vi "SLMControl.vi"(8 "error in":errorcluster, 9 "Com-in":refnum<queue>, 10 "Com-out":refnum<queue>) -> (0 "error out":errorcluster)   [LabVIEW 2013, in "SLMControl.lvlib"]
uses:
  SLMControl.lvlib
  SA-SLMAPI/Sources/Message.lvclass
  Sources/Main/Status-LEDs.ctl
  Sources/Main/Options.ctl
  Sources/Main/Main-actions.ctl
  Sources/Main/Enqueue-modes.ctl
  Sources/Main/Deposition-actions.ctl
  Sources/Main/Lasing-actions.ctl
  Sources/Main/SC-Main.lvclass
  Sources/UI/SC-UI.lvclass
panel:
  in  "Clear":bool
  in  "Load configuration":bool
  in  "Abort":bool
  in  "Save configuration":bool
  in  "Activate":bool
  in  "Load deposition files":bool
  in  "Load lasing files":bool
  in  "Execute":bool
  in  "Help":bool
  in  "Options":T1
  out "Last elapsed time":dbl caption="Time [s]" format="%.2f"
  out "Current iteration":i32
  out "Current layer":i32
  out "Lasing job":string
  out "Deposition status":string
  out "Status LEDs":T2 caption="Status"
  in  "Files":i32(listbox)
  out "Status":string caption="Status:"
  out "Action":string caption="Action:"
  # "Config"
  # "Exec"
  # "Files"
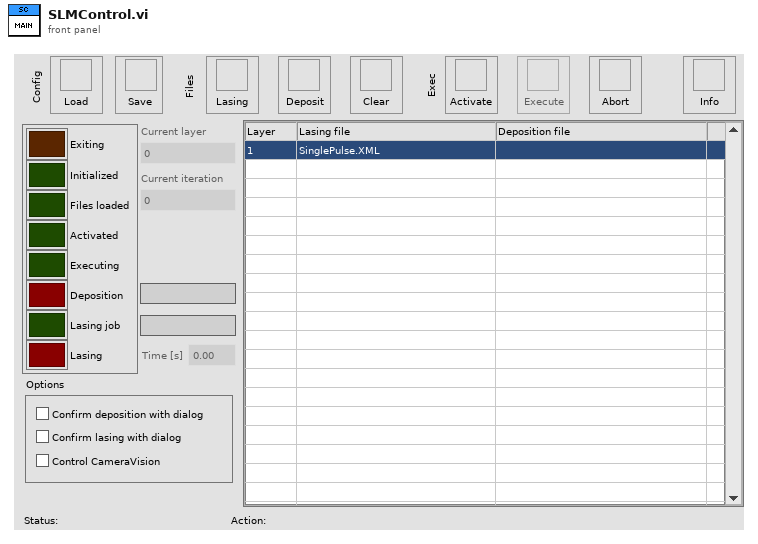
[diagram p1: front panel]
types:
  T1 = typedef "SLMControl.lvlib/SC-Main.lvclass/Options.ctl" = cluster{"Confirm deposition":bool, "Confirm lasing":bool, " Control CameraVision":bool}
  T2 = typedef "SLMControl.lvlib/SC-Main.lvclass/Status-LEDs.ctl" = cluster{"Exiting led":bool, "Initialized led":bool, "Files loaded led":bool, "Activated led":bool, "Executing led":bool, "Deposition led":bool, "Lasing job led":bool, "Lasing led":bool}
  T3 = typedef "SLMControl.lvlib/SC-Main.lvclass/Main-actions.ctl" = enum16{"Idle", "Initialize", "Load configuration", "Save configuration", "Load lasing files", "Load deposition files", "Refresh files", "Clear files", "Open lasing file", "Activate", "Start", "Start deposition cycle", "Start lasing cycle", "Iterate", "Abort", "Stop", "Exit"}
  T4 = typedef "SLMControl.lvlib/SC-Main.lvclass/Object-reference.ctl" = refnum<data-value>
  T5 = typedef "SLMControl.lvlib/SC-Main.lvclass/Enqueue-modes.ctl" = enum16{"Default", "Priority", "Flush"}
  T6 = typedef "SLMControl.lvlib/SC-Main.lvclass/Deposition-actions.ctl" = enum16{"Idle", "Activate", "Load deposition", "Launch deposition", "Wait for deposition end", "Signal lasing", "Abort", "Reset", "Exit"}
  T7 = typedef "SLMControl.lvlib/SC-Main.lvclass/Lasing-actions.ctl" = enum16{"Idle", "Activate", "Load lasing file", "Launch lasing", "Wait for lasing end", "Signal iterate", "Signal abort", "Abort", "Reset", "Exit"}
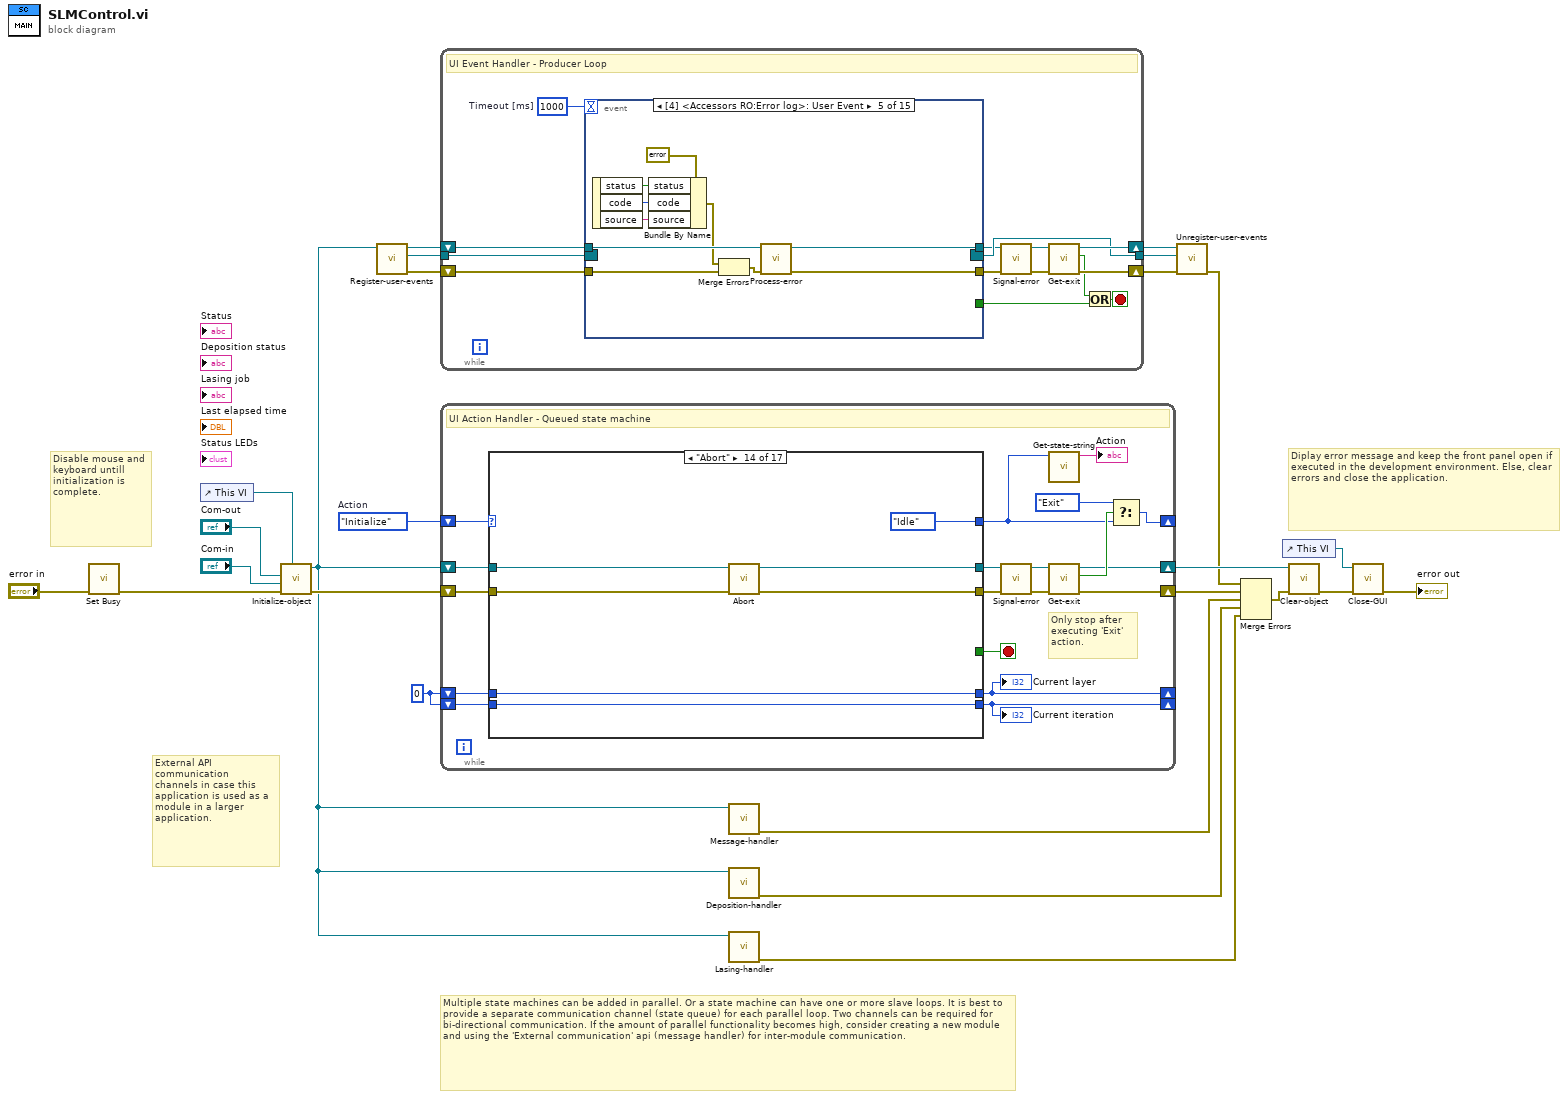
[diagram p0: block diagram]
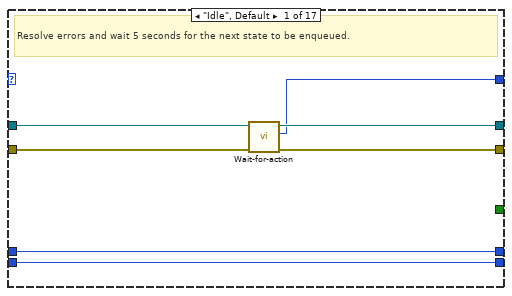
[diagram p2: hidden frame]
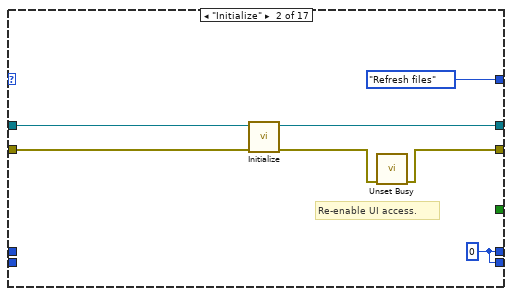
[diagram p3: hidden frame]
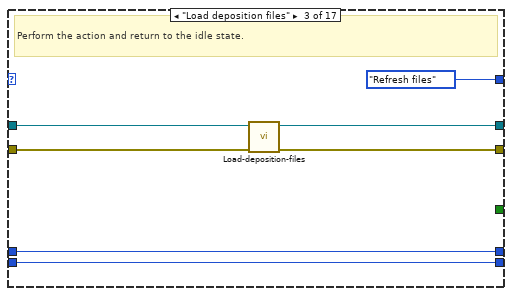
[diagram p4: hidden frame]
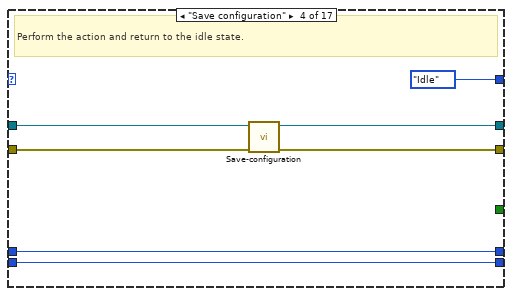
[diagram p5: hidden frame]
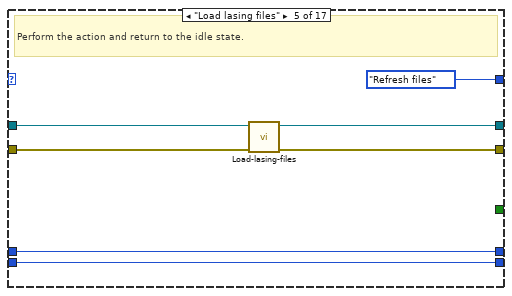
[diagram p6: hidden frame]
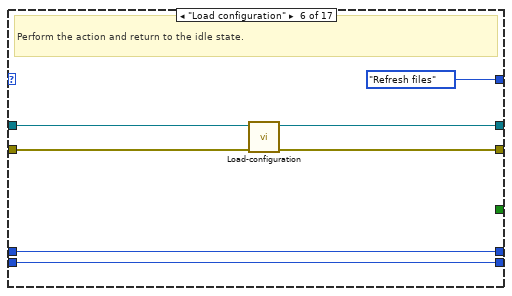
[diagram p7: hidden frame]
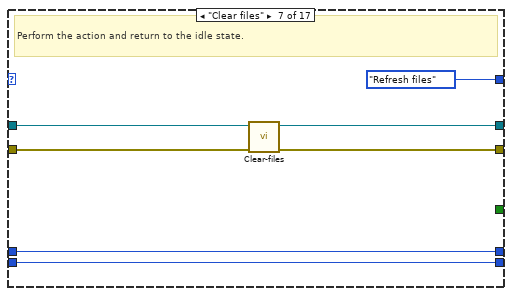
[diagram p8: hidden frame]
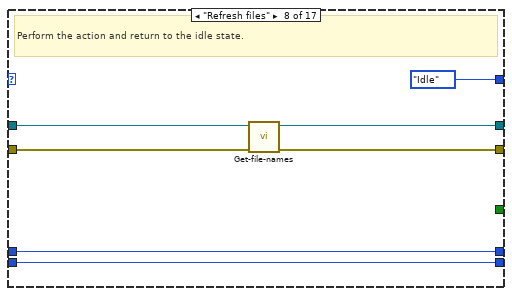
[diagram p9: hidden frame]
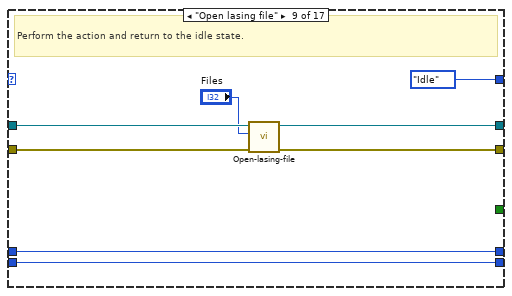
[diagram p10: hidden frame]
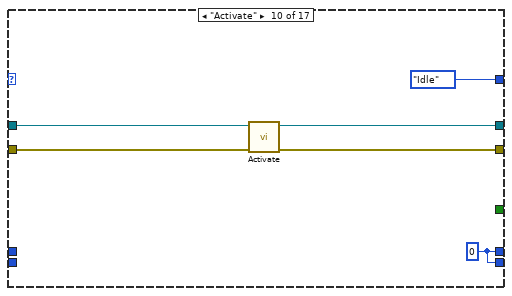
[diagram p11: hidden frame]
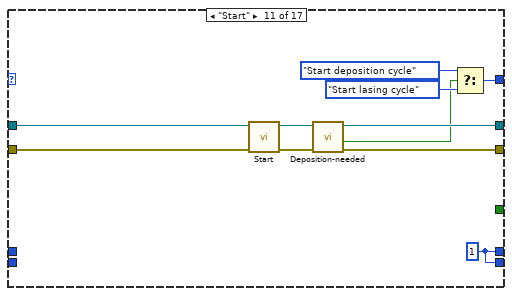
[diagram p12: hidden frame]
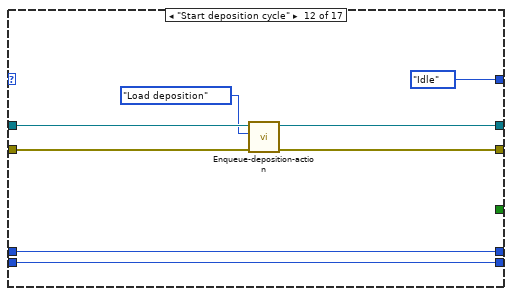
[diagram p13: hidden frame]
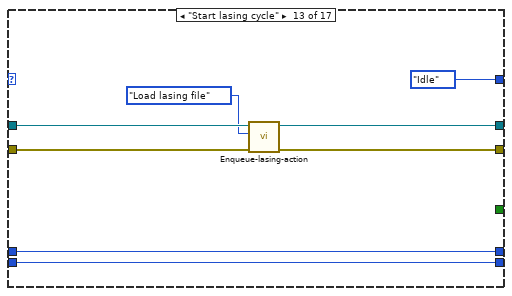
[diagram p14: hidden frame]
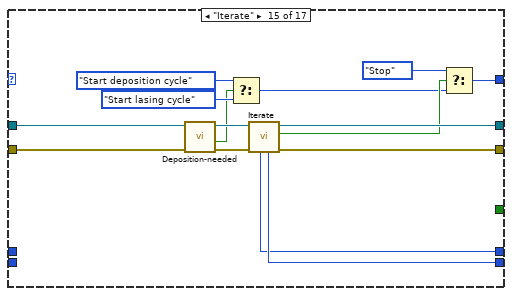
[diagram p15: hidden frame]
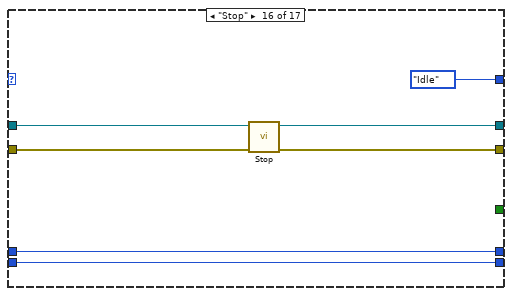
[diagram p16: hidden frame]
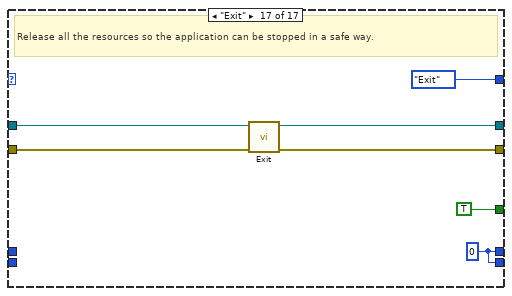
[diagram p17: hidden frame]
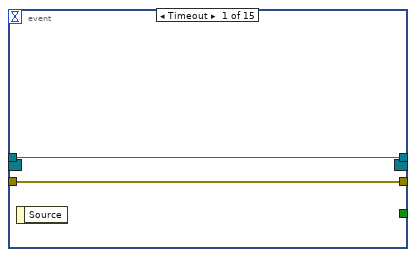
[diagram p18: hidden frame]
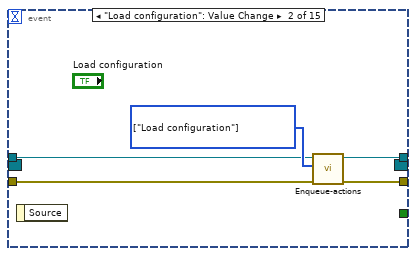
[diagram p19: hidden frame]
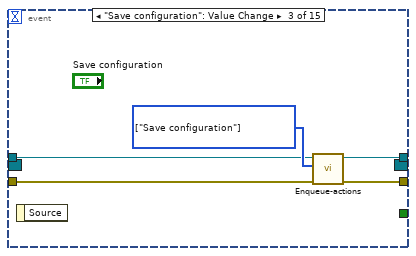
[diagram p20: hidden frame]
diagram:
  w5 = 0
  w25 = Main-actions."Initialize"  # Action
  # "External API communication\nchannels in case this application is used as a module in a larger application."
  # "Multiple state machines can be added in parallel. Or a state machine can have one or more slave loops. It is best to provide a separate communication channel (state queue) for each parallel loop. Two channels can be required for bi-directional communication. If the amount of parallel functionality becomes high, consider creating a new module and using the 'External communication' api (message handler) for inter-module communication."
  # "Disable mouse and keyboard untill initialization is complete."
  # "Diplay error message and keep the front panel open if executed in the development environment. Else, clear errors and close the application."
  n1 = call <vilib>:"Set Busy.vi"("error in (no error)"="error in") -> ("error out"=w1:errorcluster)  [unwired: 9 in, 1 out]
  n2 = control-ref of="This VI"() -> (w19:refnum<vi>)
  n3 = call "Initialize-object.vi"("Main VI ref"=w19, "error in (no error)"=w1, "Client channel"="Com-in", "Server channel"="Com-out") -> ("error out"=w17:errorcluster, "Object ref out"=w7:T4)  [unwired: 6 in]
  n4 = call "Register-user-events.vi"("Object ref in"=w7) -> ("error out"=w13:errorcluster, "Event registration"=w12:refnum<event-registration>, "Object ref out"=w14:T4)  [unwired: 8 in]
  n5 = while {
    shift-right: [w33] -> w11
    shift-left: w13 -> [w38]
    shift-right: [w34] -> w9
    shift-left: w14 -> [w37]
    tunnel: w12 -> [w32]
    tunnel: [w31] -> w8
    stop <- w28 stop-if-true
    w39 = 1000  # Timeout [ms]
    # "UI Event Handler - Producer Loop"
    n6 = event shown="[4] <Accessors RO:Error log>: User Event" {
      selector: w32 -> [_ _ _ _ _ _ _ _ _ _ _ _ _ _ _]
      dyn-events: [_ _ _ _ _ _ _ _ _ _ _ _ _ _ _] -> w31
      timeout: w39 -> [_ _ _ _ _ _ _ _ _ _ _ _ _ _ _]
      tunnel: w38 -> [w41 w46 w51 w56 w64 w71 w76 w79 w86 w91 w96 w102 w105 w107 w109]
      tunnel: [w41 w45 w50 w55 w63 w70 w75 w80 w85 w90 w95 w101 w105 w107 w114] -> w29
      tunnel: w37 -> [w40 w43 w48 w53 w66 w68 w73 w78 w84 w88 w93 w99 w103 w106 w110]
      tunnel: [w40 w42 w47 w52 w65 w67 w72 w81 w83 w87 w92 w98 w103 w106 w111] -> w30
      tunnel: [_ _ _ _ _ _ _ _ _ _ _ _ _ _ TRUE] -> w26
      event Timeout {
        n7 = event-data() -> ()  [unwired: 1 in, 1 out]
      }
      event "Load configuration": Value Change {
        w44 = T3[] [enum."Load configuration"] items=["Idle", "Initialize", "Load configuration", "Save configuration", "Load lasing files", "Load deposition files", "Refresh files", "Clear files", "Open lasing file", "Activate", "Start", "Start deposition cycle", "Start lasing cycle", "Iterate", "Abort", "Stop", "Exit"] ("State array")
        n8 = event-data() -> ()  [unwired: 1 in, 1 out]
        n9 = call "Enqueue-actions.vi"("error in (no error)"=w46, "State array"=w44, "State queue in"=w43) -> ("error out"=w45:errorcluster, "State queue out"=w42:T4)  [unwired: 6 in, 1 out]
      }
      event "Save configuration": Value Change {
        w49 = T3[] [enum."Save configuration"] items=["Idle", "Initialize", "Load configuration", "Save configuration", "Load lasing files", "Load deposition files", "Refresh files", "Clear files", "Open lasing file", "Activate", "Start", "Start deposition cycle", "Start lasing cycle", "Iterate", "Abort", "Stop", "Exit"] ("State array")
        n10 = event-data() -> ()  [unwired: 1 in, 1 out]
        n11 = call "Enqueue-actions.vi"("error in (no error)"=w51, "State array"=w49, "State queue in"=w48) -> ("error out"=w50:errorcluster, "State queue out"=w47:T4)  [unwired: 6 in, 1 out]
      }
      event "Load lasing files": Value Change {
        w54 = T3[] [enum."Load lasing files"] items=["Idle", "Initialize", "Load configuration", "Save configuration", "Load lasing files", "Load deposition files", "Refresh files", "Clear files", "Open lasing file", "Activate", "Start", "Start deposition cycle", "Start lasing cycle", "Iterate", "Abort", "Stop", "Exit"] ("State array")
        n12 = event-data() -> ()  [unwired: 1 in, 1 out]
        n13 = call "Enqueue-actions.vi"("error in (no error)"=w56, "State array"=w54, "State queue in"=w53) -> ("error out"=w55:errorcluster, "State queue out"=w52:T4)  [unwired: 6 in, 1 out]
      }
      event User Event {
        n14 = event-data() -> ("status"=w61:bool, "code"=w60:i32, "source"=w59:string)  [unwired: 1 in]
        n15 = Bundle By Name(cluster=errorcluster {"status"=FALSE, "code"=0, "source"=""} ("error constant"), "status"=w61, "code"=w60, "source"=w59) -> (w57:errorcluster)
        n16 = Merge Errors(w57, w64) -> (w58:errorcluster)
        n17 = call "Process-error.vi"("error in (no error)"=w58, "Data in"=w66) -> ("error out"=w63:errorcluster, "Data out"=w65:T4)  [unwired: 8 in]
      }
      event "Load deposition files": Value Change {
        w69 = T3[] [enum."Load deposition files"] items=["Idle", "Initialize", "Load configuration", "Save configuration", "Load lasing files", "Load deposition files", "Refresh files", "Clear files", "Open lasing file", "Activate", "Start", "Start deposition cycle", "Start lasing cycle", "Iterate", "Abort", "Stop", "Exit"] ("State array")
        n18 = event-data() -> ()  [unwired: 1 in, 1 out]
        n19 = call "Enqueue-actions.vi"("error in (no error)"=w71, "State array"=w69, "State queue in"=w68) -> ("error out"=w70:errorcluster, "State queue out"=w67:T4)  [unwired: 6 in, 1 out]
      }
      event "Clear": Value Change {
        w74 = T3[] [enum."Clear files"] items=["Idle", "Initialize", "Load configuration", "Save configuration", "Load lasing files", "Load deposition files", "Refresh files", "Clear files", "Open lasing file", "Activate", "Start", "Start deposition cycle", "Start lasing cycle", "Iterate", "Abort", "Stop", "Exit"] ("State array")
        n20 = event-data() -> ()  [unwired: 1 in, 1 out]
        n21 = call "Enqueue-actions.vi"("error in (no error)"=w76, "State array"=w74, "State queue in"=w73) -> ("error out"=w75:errorcluster, "State queue out"=w72:T4)  [unwired: 6 in, 1 out]
      }
      event Value Change {
        n22 = event-data() -> ()  [unwired: 1 in, 2 out]
        n23 = call "Set-options.vi"("error in (no error)"=w79, "Options"="Options", "Object ref in"=w78) -> ("error out"=w80:errorcluster, "Object ref out"=w81:T4)  [unwired: 7 in]
      }
      event "Files": Double Click {
        w82 = T3[] [enum."Open lasing file"] items=["Idle", "Initialize", "Load configuration", "Save configuration", "Load lasing files", "Load deposition files", "Refresh files", "Clear files", "Open lasing file", "Activate", "Start", "Start deposition cycle", "Start lasing cycle", "Iterate", "Abort", "Stop", "Exit"] ("State array")
        n24 = event-data() -> ()  [unwired: 1 in, 2 out]
        n25 = call "Enqueue-actions.vi"("error in (no error)"=w86, "State array"=w82, "State queue in"=w84) -> ("error out"=w85:errorcluster, "State queue out"=w83:T4)  [unwired: 6 in, 1 out]
      }
      event "Activate": Value Change {
        w89 = T3[] [enum."Activate"] items=["Idle", "Initialize", "Load configuration", "Save configuration", "Load lasing files", "Load deposition files", "Refresh files", "Clear files", "Open lasing file", "Activate", "Start", "Start deposition cycle", "Start lasing cycle", "Iterate", "Abort", "Stop", "Exit"] ("State array")
        n26 = event-data() -> ()  [unwired: 1 in, 1 out]
        n27 = call "Enqueue-actions.vi"("error in (no error)"=w91, "State array"=w89, "State queue in"=w88) -> ("error out"=w90:errorcluster, "State queue out"=w87:T4)  [unwired: 6 in, 1 out]
      }
      event "Execute": Value Change {
        w94 = T3[] [enum."Start"] items=["Idle", "Initialize", "Load configuration", "Save configuration", "Load lasing files", "Load deposition files", "Refresh files", "Clear files", "Open lasing file", "Activate", "Start", "Start deposition cycle", "Start lasing cycle", "Iterate", "Abort", "Stop", "Exit"] ("State array")
        n28 = event-data() -> ()  [unwired: 1 in, 1 out]
        n29 = call "Enqueue-actions.vi"("error in (no error)"=w96, "State array"=w94, "State queue in"=w93) -> ("error out"=w95:errorcluster, "State queue out"=w92:T4)  [unwired: 6 in, 1 out]
      }
      event "Abort": Value Change {
        w100 = T3[] [enum."Abort"] items=["Idle", "Initialize", "Load configuration", "Save configuration", "Load lasing files", "Load deposition files", "Refresh files", "Clear files", "Open lasing file", "Activate", "Start", "Start deposition cycle", "Start lasing cycle", "Iterate", "Abort", "Stop", "Exit"] ("State array")
        n30 = event-data() -> ()  [unwired: 1 in, 1 out]
        n31 = call "Enqueue-actions.vi"("Enqueue mode"=Enqueue-modes."Flush", "error in (no error)"=w102, "State array"=w100, "State queue in"=w99) -> ("error out"=w101:errorcluster, "State queue out"=w98:T4)  [unwired: 5 in, 1 out]
      }
      event "Help": Value Change {
        # "Toggle the visibility of the context help window."
        n32 = event-data() -> ()  [unwired: 1 in, 1 out]
        n33 = Control Help Window(1:"Help") -> ()  [unwired: 1 in]
      }
      event Menu Selection (User) {
        n34 = event-data() -> ()  [unwired: 1 in, 2 out]
      }
      event Panel Close? {
        w112 = T3[] [enum."Abort", enum."Exit"] items=["Idle", "Initialize", "Load configuration", "Save configuration", "Load lasing files", "Load deposition files", "Refresh files", "Clear files", "Open lasing file", "Activate", "Start", "Start deposition cycle", "Start lasing cycle", "Iterate", "Abort", "Stop", "Exit"] ("State array")
        # "Discard event, to allow time to exit in a safe way."
        # "The user can stop the program by pressing the X in the window corner."
        n35 = event-data() -> ()  [unwired: 1 in, 1 out]
        n36 = call "Enqueue-actions.vi"("Enqueue mode"=Enqueue-modes."Flush", "error in (no error)"=w109, "State array"=w112, "State queue in"=w110) -> ("error out"=w114:errorcluster, "State queue out"=w111:T4)  [unwired: 5 in, 1 out]
        n37 = event-data("Discard?"=TRUE ("Exit?")) -> ()  [unwired: 1 in, 1 out]
      }
    }
    n38 = call "Signal-error.vi"("error in (no error)"=w29, "Data in"=w30) -> ("error out"=w36:errorcluster, "Data out"=w35:T4)  [unwired: 8 in]
    n39 = call "Get-exit.vi"("error in (no error)"=w36, "Object ref in"=w35) -> ("error out"=w33:errorcluster, "Exit?"=w27:bool, "Object ref out"=w34:T4)  [unwired: 7 in]
    n40 = Or(x=w27, y=w26) -> (x .or. y?=w28:bool)
  }
  n41 = while {
    shift-right: [w128] -> _
    shift-left: w25 -> [w131]
    shift-right: [w122] -> w18
    shift-left: w7 -> [w133]
    shift-right: [w121] -> w24
    shift-left: w17 -> [w132]
    shift-right: [w117] -> _
    shift-left: w5 -> [w120]
    shift-right: [w118] -> _
    shift-left: w5 -> [w119]
    stop <- w134 stop-if-true
    # "Only stop after executing 'Exit' action."
    # "UI Action Handler - Queued state machine"
    n42 = case shown="\"Abort\"" w131 {
      tunnel: [w138 Main-actions."Refresh files" ("States") Main-actions."Refresh files" ("States") Main-actions."Idle" ("States") Main-actions."Refresh files" ("States") Main-actions."Refresh files" ("States") Main-actions."Refresh files" ("States") Main-actions."Idle" ("States") Main-actions."Idle" ("States") Main-actions."Idle" ("States") w207 Main-actions."Idle" ("States") Main-actions."Idle" ("States") Main-actions."Idle" ("States") w251 Main-actions."Idle" ("States") Main-actions."Exit" ("States")] -> w125
      tunnel: [_ _ _ _ _ _ _ _ _ _ _ _ _ _ _ _ TRUE] -> w134
      tunnel: w133 -> [w140 w146 w154 w161 w168 w175 w182 w189 w197 w203 w215 w222 w230 w237 w246 w259 w264]
      tunnel: [w139 w145 w153 w160 w167 w174 w181 w188 w196 w202 w210 w220 w228 w235 w253 w257 w261] -> w123
      tunnel: w132 -> [w137 w144 w152 w159 w166 w173 w180 w187 w195 w200 w214 w221 w229 w236 w245 w258 w263]
      tunnel: [w141 w147 w151 w158 w165 w172 w179 w186 w194 w201 w209 w219 w227 w234 w252 w256 w262] -> w124
      tunnel: [w136 w142 w150 w157 w164 w171 w178 w185 w192 w199 w213 w217 w225 w233 w247 w255 w265] -> w117
      tunnel: w120 -> [w136 _ w150 w157 w164 w171 w178 w185 w192 _ _ w217 w225 w233 _ w255 _]
      tunnel: w119 -> [w135 _ w149 w156 w163 w170 w177 w184 w191 _ _ w216 w224 w232 _ w254 _]
      tunnel: [w135 w142 w149 w156 w163 w170 w177 w184 w191 w199 w213 w216 w224 w232 w248 w254 w265] -> w118
      frame "Idle", Default {
        # "Resolve errors and wait 5 seconds for the next state to be enqueued."
        n43 = call "Wait-for-action.vi"("error in (no error)"=w137, "Object ref in"=w140) -> ("error out"=w141:errorcluster, "Next action"=w138:T3, "Object ref out"=w139:T4)  [unwired: 7 in]
      }
      frame "Initialize" {
        w142 = 0
        # "Re-enable UI access."
        n44 = call "Initialize.vi"("error in (no error)"=w144, "Object ref in"=w146) -> ("error out"=w143:errorcluster, "Object ref out"=w145:T4)  [unwired: 8 in]
        n45 = call <vilib>:"Unset Busy.vi"("error in (no error)"=w143) -> ("error out"=w147:errorcluster)  [unwired: 10 in]
      }
      frame "Load deposition files" {
        # "Perform the action and return to the idle state."
        n46 = call "Load-deposition-files.vi"("error in (no error)"=w152, "Object ref in"=w154) -> ("error out"=w151:errorcluster, "Object ref out"=w153:T4)  [unwired: 8 in]
      }
      frame "Save configuration" {
        # "Perform the action and return to the idle state."
        n47 = call "Save-configuration.vi"("error in (no error)"=w159, "Object ref in"=w161) -> ("error out"=w158:errorcluster, "Object ref out"=w160:T4)  [unwired: 7 in, 1 out]
      }
      frame "Load lasing files" {
        # "Perform the action and return to the idle state."
        n48 = call "Load-lasing-files.vi"("error in (no error)"=w166, "Object ref in"=w168) -> ("error out"=w165:errorcluster, "Object ref out"=w167:T4)  [unwired: 8 in]
      }
      frame "Load configuration" {
        # "Perform the action and return to the idle state."
        n49 = call "Load-configuration.vi"("error in (no error)"=w173, "Object ref in"=w175) -> ("error out"=w172:errorcluster, "Object ref out"=w174:T4)  [unwired: 8 in]
      }
      frame "Clear files" {
        # "Perform the action and return to the idle state."
        n50 = call "Clear-files.vi"("error in (no error)"=w180, "Object ref in"=w182) -> ("error out"=w179:errorcluster, "Object ref out"=w181:T4)  [unwired: 8 in]
      }
      frame "Refresh files" {
        # "Perform the action and return to the idle state."
        n51 = call "Get-file-names.vi"("error in (no error)"=w187, "Object ref in"=w189) -> ("error out"=w186:errorcluster, "Object ref out"=w188:T4)  [unwired: 7 in, 1 out]
      }
      frame "Open lasing file" {
        # "Perform the action and return to the idle state."
        n52 = call "Open-lasing-file.vi"("error in (no error)"=w195, "File index"="Files", "Object ref in"=w197) -> ("error out"=w194:errorcluster, "Object ref out"=w196:T4)  [unwired: 6 in, 1 out]
      }
      frame "Activate" {
        w199 = 0
        n53 = call "Activate.vi"("error in (no error)"=w200, "Object ref in"=w203) -> ("error out"=w201:errorcluster, "Object ref out"=w202:T4)  [unwired: 8 in]
      }
      frame "Start" {
        w213 = 1
        n54 = call "Start.vi"("error in (no error)"=w214, "Object ref in"=w215) -> ("error out"=w211:errorcluster, "Object ref out"=w212:T4)  [unwired: 8 in]
        n55 = call "Deposition-needed.vi"("error in (no error)"=w211, "Object ref in"=w212) -> ("error out"=w209:errorcluster, "Deposit?"=w205:bool, "Object ref out"=w210:T4)  [unwired: 7 in]
        n56 = Select(t=Main-actions."Start deposition cycle" ("States"), s=w205, f=Main-actions."Start lasing cycle" ("States")) -> (s? t:f=w207:T3)
      }
      frame "Start deposition cycle" {
        n57 = call "Enqueue-deposition-action.vi"("error in (no error)"=w221, "Action"=Deposition-actions."Load deposition" ("Execution action"), "State queue in"=w222) -> ("error out"=w219:errorcluster, "State queue out"=w220:T4)  [unwired: 6 in, 1 out]
      }
      frame "Start lasing cycle" {
        n58 = call "Enqueue-lasing-action.vi"("error in (no error)"=w229, "Action"=Lasing-actions."Load lasing file" ("Execution action"), "State queue in"=w230) -> ("error out"=w227:errorcluster, "State queue out"=w228:T4)  [unwired: 6 in, 1 out]
      }
      frame "Abort" {
        n59 = call "Abort.vi"("error in (no error)"=w236, "Object ref in"=w237) -> ("error out"=w234:errorcluster, "Object ref out"=w235:T4)  [unwired: 8 in]
      }
      frame "Iterate" {
        n60 = call "Deposition-needed.vi"("error in (no error)"=w245, "Object ref in"=w246) -> ("error out"=w244:errorcluster, "Deposit?"=w240:bool, "Object ref out"=w243:T4)  [unwired: 7 in]
        n61 = Select(t=Main-actions."Start deposition cycle" ("f"), s=w240, f=Main-actions."Start lasing cycle") -> (s? t:f=w239:T3)
        n62 = call "Iterate.vi"("error in (no error)"=w244, "Object ref in"=w243) -> ("error out"=w252:errorcluster, "Finished?"=w249:bool, "Object ref out"=w253:T4, "Current iteration"=w248:i32, "Current layer"=w247:i32)  [unwired: 5 in]
        n63 = Select(t=Main-actions."Stop" ("States"), s=w249, f=w239) -> (s? t:f=w251:T3)
      }
      frame "Stop" {
        n64 = call "Stop.vi"("error in (no error)"=w258, "Object ref in"=w259) -> ("error out"=w256:errorcluster, "Object ref out"=w257:T4)  [unwired: 8 in]
      }
      frame "Exit" {
        w265 = 0
        # "Release all the resources so the application can be stopped in a safe way."
        n65 = call "Exit.vi"("error in (no error)"=w263, "Object ref in"=w264) -> ("error out"=w262:errorcluster, "Object ref out"=w261:T4)  [unwired: 8 in]
      }
    }
    "Current layer" <- w117
    "Current iteration" <- w118
    n66 = call "Signal-error.vi"("error in (no error)"=w124, "Data in"=w123) -> ("error out"=w130:errorcluster, "Data out"=w129:T4)  [unwired: 8 in]
    n67 = call "Get-state-string.vi"("States"=w125) -> ("State string"=→"Action":string)  [unwired: 10 in]
    n68 = call "Get-exit.vi"("error in (no error)"=w130, "Object ref in"=w129) -> ("error out"=w121:errorcluster, "Exit?"=w126:bool, "Object ref out"=w122:T4)  [unwired: 7 in]
    n69 = Select(t=Main-actions."Exit" ("States"), s=w126, f=w125) -> (s? t:f=w128:T3)
  }
  n70 = call "Message-handler.vi"("PD in"=w7) -> ("error out"=w16:errorcluster)  [unwired: 9 in, 1 out]
  n71 = call "Deposition-handler.vi"("Object ref in"=w7) -> ("error out"=w15:errorcluster)  [unwired: 9 in, 1 out]
  n72 = call "Lasing-handler.vi"("Object ref in"=w7) -> ("error out"=w6:errorcluster)  [unwired: 9 in, 1 out]
  n73 = call "Unregister-user-events.vi"("error in (no error)"=w11, "Event registration"=w8, "Object ref in"=w9) -> ("error out"=w10:errorcluster)  [unwired: 7 in, 1 out]
  n74 = Merge Errors(w10, w24, w16, w15, w6) -> (w22:errorcluster)
  n75 = control-ref of="This VI"() -> (w2:refnum<vi>)
  n76 = call "Clear-object.vi"("error in (no error)"=w22, "Object ref in"=w18) -> ("error out"=w21:errorcluster)  [unwired: 9 in]
  n77 = call "Close-GUI.vi"("error in (no error)"=w21, "Main VI"=w2) -> ("error out"=→"error out":errorcluster)  [unwired: 9 in]
